vi "Subscribe.vi"   [LabVIEW 2020, in "wamplv.lvlib" / "WAMP Client.lvclass"]
uses:
  WAMP Client.lvclass
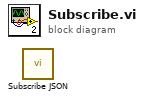
[diagram p0: block diagram]
diagram:
  n1 = call-dynamic "Subscribe JSON.vi"() -> ()  [unwired: 7 in, 5 out]
